vi "Command Robot.vi"(11 "all rows":dbl[][](array[numeric])) -> ()   [LabVIEW 2020]
uses:
  Framework/Robot Global Data.vi
panel:
  out "X-DriveAuto":dbl
  out "Y-DriveAuto":dbl
  out "Transfer Release":bool
  out "Transfer Up":bool
  out "Intake":bool
  out "Shooter":bool
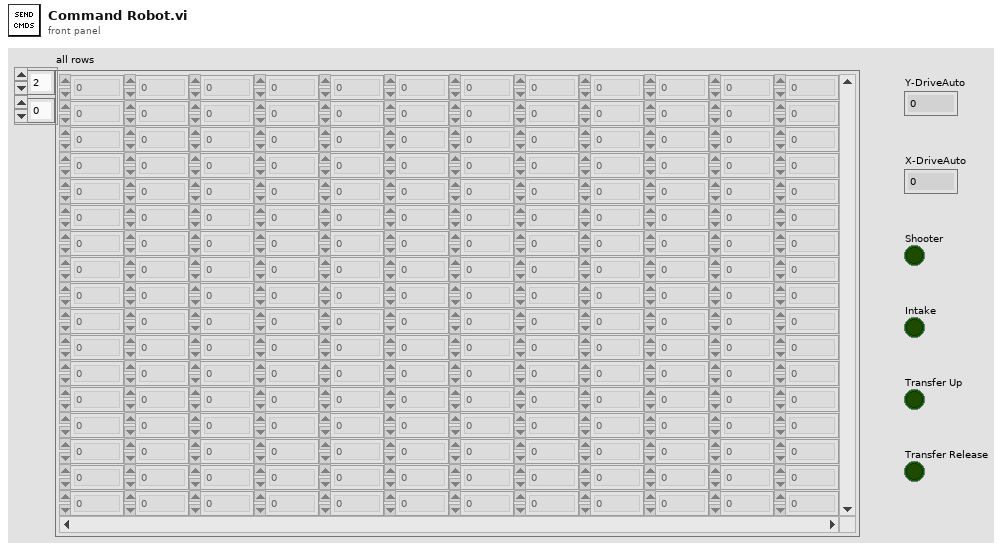
[diagram p1: front panel]
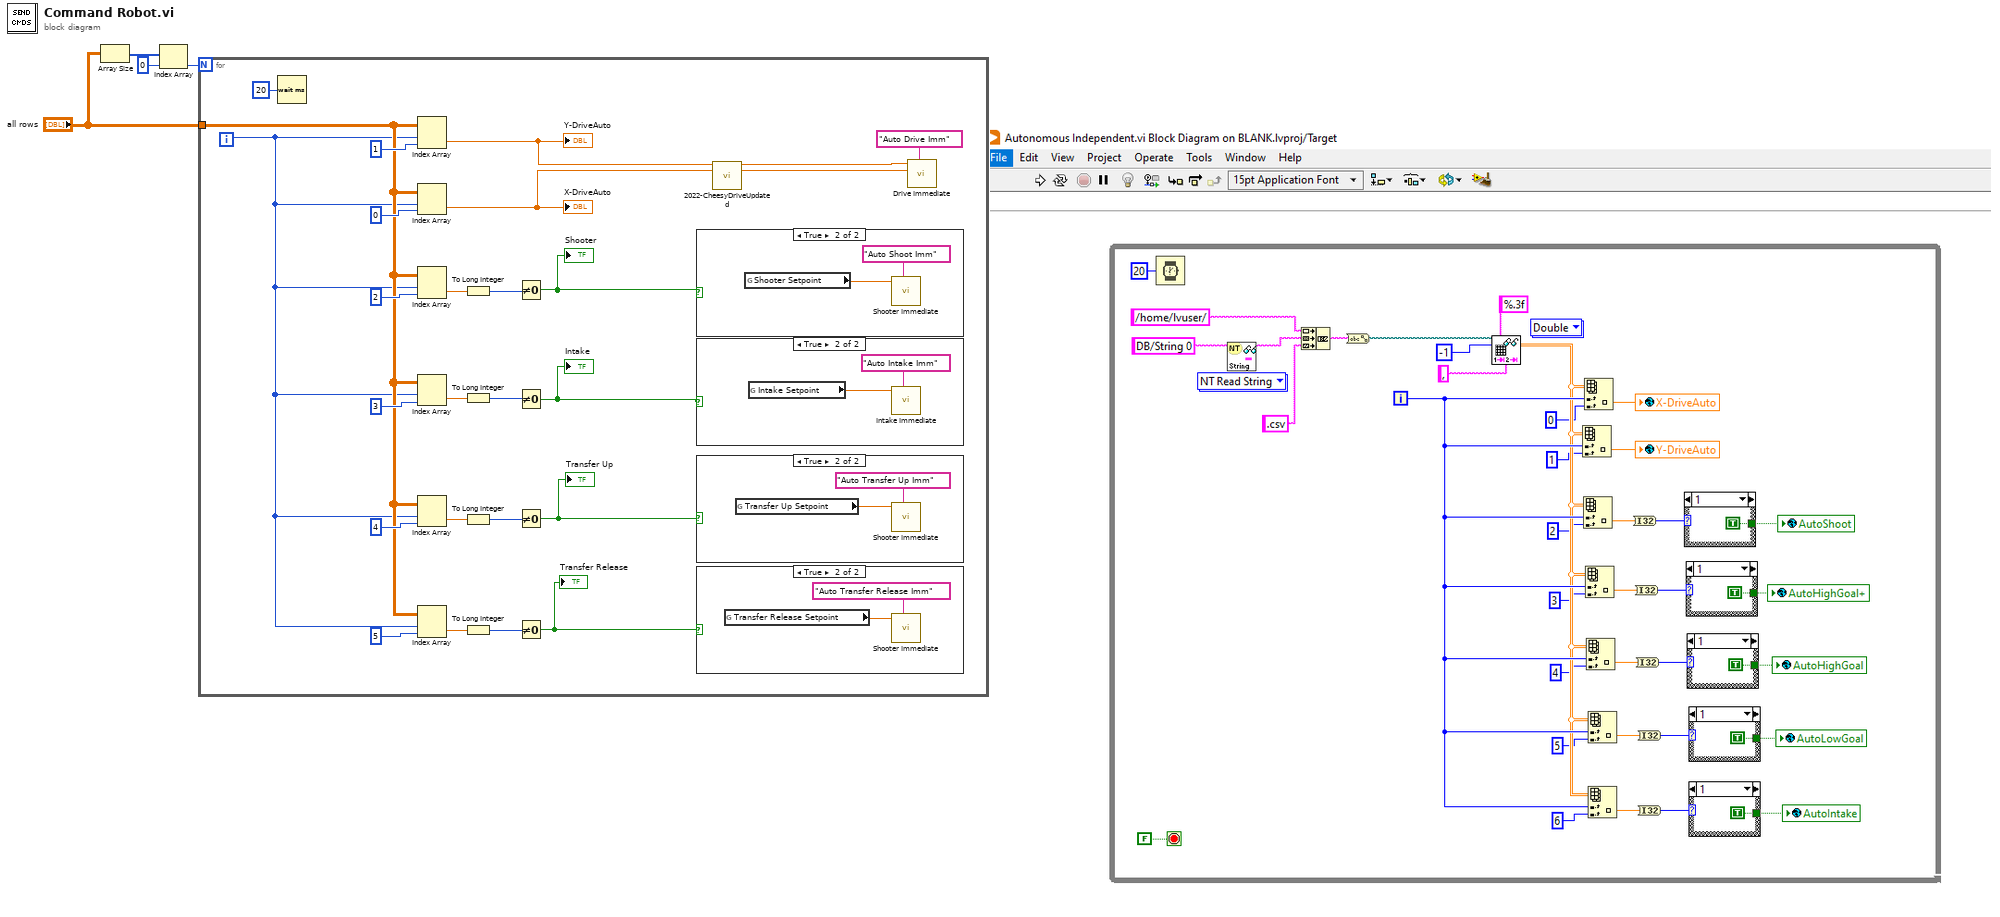
[diagram p0: block diagram]
diagram:
  n1 = Array Size(array="all rows") -> (size(s)=w2:i32[])
  n2 = Index Array(array=w2, index=0) -> (element=w1:i32)
  n3 = for {
    N: w1 -> [_]
    tunnel: "all rows" -> [w20]
    i -> [w19]
    n4 = Wait (ms)(milliseconds to wait=u32 20) -> ()  [unwired: 1 out]
    n5 = Index Array(array=w20, index (row)=w19, index (col)=1 ("disabled index (col)")) -> (element=w10:dbl)
    "Y-DriveAuto" <- w10
    n6 = Index Array(array=w20, index (row)=w19, index (col)=0 ("disabled index (col)")) -> (element=w9:dbl)
    "X-DriveAuto" <- w9
    n7 = Index Array(array=w20, index (row)=w19, index (col)=2 ("disabled index (col)")) -> (element=w24:dbl)
    n8 = Index Array(array=w20, index (row)=w19, index (col)=3 ("disabled index (col)")) -> (element=w26:dbl)
    n9 = Index Array(array=w20, index (row)=w19, index (col)=4 ("disabled index (col)")) -> (element=w28:dbl)
    n10 = Index Array(array=w20, index (row)=w19, index (col)=5 ("disabled index (col)")) -> (element=w30:dbl)
    n11 = To Long Integer(number=w24) -> (32bit integer=w18:i32)
    n12 = To Long Integer(number=w26) -> (32bit integer=w17:i32)
    n13 = To Long Integer(number=w28) -> (32bit integer=w16:i32)
    n14 = To Long Integer(number=w30) -> (32bit integer=w15:i32)
    n15 = Not Equal To 0?(x=w18) -> (x != 0?=w8:bool)
    "Shooter" <- w8
    n16 = Not Equal To 0?(x=w17) -> (x != 0?=w7:bool)
    "Intake" <- w7
    n17 = Not Equal To 0?(x=w16) -> (x != 0?=w6:bool)
    "Transfer Up" <- w6
    n18 = Not Equal To 0?(x=w15) -> (x != 0?=w5:bool)
    "Transfer Release" <- w5
    n19 = case shown="True" w8 {
      frame False {
      }
      frame True {
        n20 = global read "Robot Global Data.vi" "Shooter Setpoint"() -> (w37:dbl)
        n21 = call "Shooter Immediate.vi"("Description"="Auto Shoot Imm", "Setpoint"=w37) -> ()  [unwired: 9 in, 1 out]
      }
    }
    n22 = case shown="True" w7 {
      frame False {
      }
      frame True {
        n23 = global read "Robot Global Data.vi" "Intake Setpoint"() -> (w35:dbl)
        n24 = call "Intake Immediate.vi"("Description"="Auto Intake Imm", "Setpoint"=w35) -> ()  [unwired: 9 in, 1 out]
      }
    }
    n25 = case shown="True" w6 {
      frame False {
      }
      frame True {
        n26 = global read "Robot Global Data.vi" "Transfer Up Setpoint"() -> (w33:dbl)
        n27 = call "Shooter Immediate.vi"("Description"="Auto Transfer Up Imm", "Setpoint"=w33) -> ()  [unwired: 9 in, 1 out]
      }
    }
    n28 = case shown="True" w5 {
      frame False {
      }
      frame True {
        n29 = global read "Robot Global Data.vi" "Transfer Release Setpoint"() -> (w31:dbl)
        n30 = call "Shooter Immediate.vi"("Description"="Auto Transfer Release Imm", "Setpoint"=w31) -> ()  [unwired: 9 in, 1 out]
      }
    }
    n31 = call "2022-CheesyDriveUpdated.vi"("Throttle"=w10, "Wheel"=w9) -> ("Left PWM"=w12:dbl, "Right PWM"=w13:dbl)  [unwired: 11 in, 1 out]
    n32 = call "Drive Immediate.vi"("Description"="Auto Drive Imm", "Right Setpoint"=w13, "Left Setpoint"=w12) -> ()  [unwired: 8 in, 1 out]
  }
